vi "PID Veering.vi"(6 "Deviation":dbl, 7 "Current Distance":dbl=15.0 format="%#_13g", 8 "error in (no error)":errorcluster, 11 "Refnum's":T1={"Gyro"="Gyro", "Mtr 1"="LeftMtr", "Mtr 2"="RightMtr"}) -> (0 "error out":errorcluster)   [LabVIEW 2017]
uses:
  <vilib>/addons/control/pid/pid.llb/PID (DBL).vi
  <vilib>/addons/control/pid/NI_PID_pid.lvlib
panel:
  out "Right":dbl
  out "Left":dbl
  in  "V-D":dbl format="%#_13g"
  in  "V-I":dbl format="%#_13g"
  in  "V-P":dbl=0.01 format="%#_13g"
  in  "D-D":dbl format="%#_13g"
  in  "D-I":dbl format="%#_13g"
  in  "D-P":dbl=0.02 format="%#_13g"
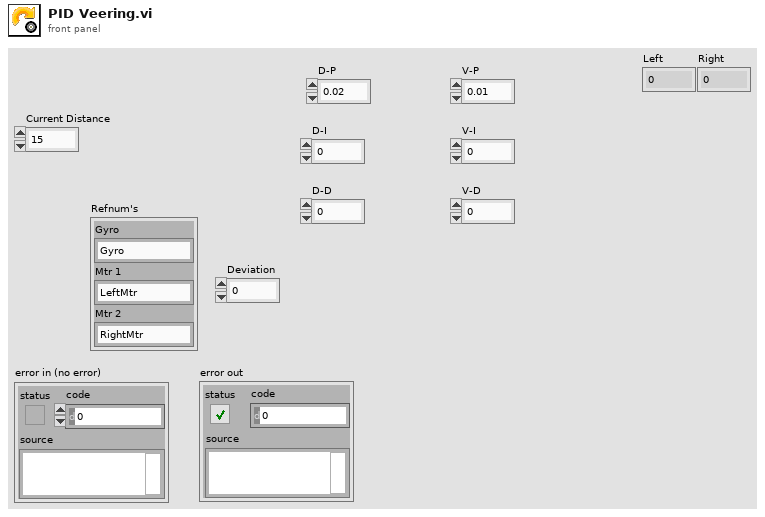
[diagram p1: front panel]
types:
  T1 = cluster{"Gyro":string, "Mtr 1":string, "Mtr 2":string}
  T2 = typedef "WPI_MotorControlDeviceRef.ctl" = cluster{"DeviceStatus":errorcluster, "Type":T3, "PWM":cluster{"PWM Channel":T4, "DeadBand":T5}, "CAN":cluster{"Device Number":u8, "SetOutput VI Ref":variant, "GetOutput VI Ref":variant, "Enable VI Ref":variant, "Disable VI Ref":variant, "Data":variant}, "Invert":bool, "DIO PWM":cluster{"PWM \"Enable\" Channel":T4, "DIOChannel":T6, "PWM Rate":dbl}}
  T3 = typedef "WPI_MotorControlType.ctl" = enum16{"PWM", "CAN", "DIO PWM"}
  T4 = typedef "FPGA_DIOPWMChannel.ctl" = enum8{"PWM 0", "PWM 1", "PWM 2", "PWM 3", "PWM 4", "PWM 5", "PWM 6", "PWM 7", "PWM 8", "PWM 9", "PWM MXP 0", "PWM MXP 1", "PWM MXP 2", "PWM MXP 3", "PWM MXP 4", "PWM MXP 5", "PWM MXP 6", "PWM MXP 7", "PWM MXP 8", "PWM MXP 9", "Invalid"}
  T5 = typedef "WPI_PWMDeadband.ctl" = cluster{"Name":string, "maxPositivePwm":i32, "minPositivePwm":i32, "centerPwm":i32, "maxNegativePwm":i32, "minNegativePwm":i32, "angularRange":u16}
  T6 = typedef "FPGA_DIOChannel.ctl" = enum8{"DIO 0", "DIO 1", "DIO 2", "DIO 3", "DIO 4", "DIO 5", "DIO 6", "DIO 7", "DIO 8", "DIO 9", "DIO MXP 0", "DIO MXP 1", "DIO MXP 2", "DIO MXP 3", "DIO MXP 4", "DIO MXP 5", "DIO MXP 6", "DIO MXP 7", "DIO MXP 8", "DIO MXP 9", "DIO MXP 10", "DIO MXP 11", "DIO MXP 12", "DIO MXP 13", "DIO MXP 14", "DIO MXP 15", "SPI Port CS1", "SPI Port CS2", "SPI Port CS3", "SPI Port MISO", "SPI Port MOSI", "Invalid"}
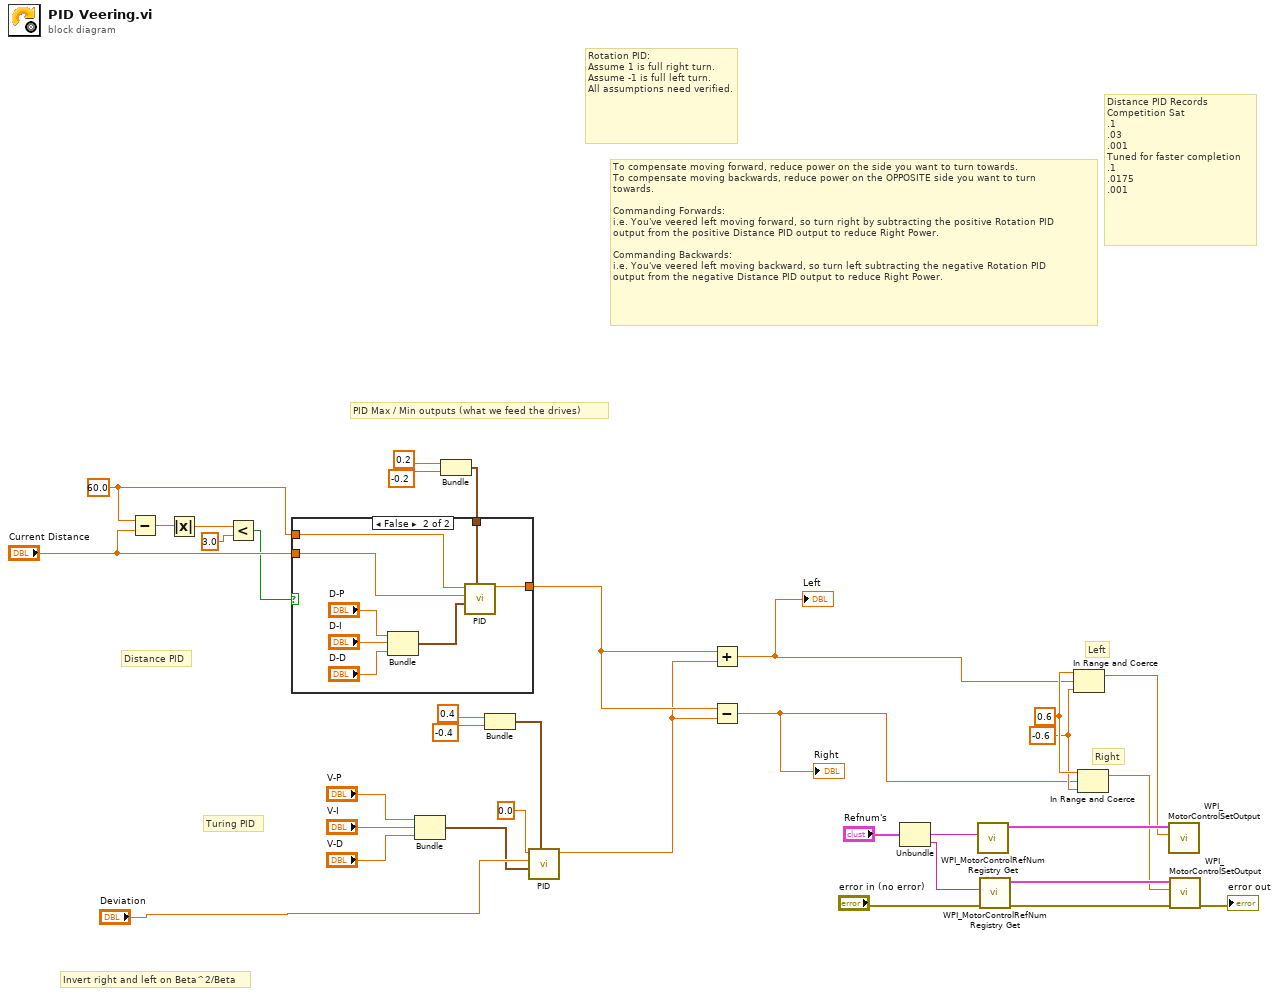
[diagram p0: block diagram]
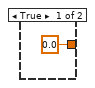
[diagram p2: hidden frame]
diagram:
  w13 = 60.0 ("setpoint")
  w28 = -0.6
  w29 = 0.6
  # "Right"
  # "Left"
  # "Turing PID"
  # "Distance PID"
  # "Distance PID Records\nCompetition Sat\n.1\n.03\n.001\nTuned for faster completion\n.1\n.0175\n.001"
  # "Invert right and left on Beta^2/Beta"
  # "To compensate moving forward, reduce power on the side you want to turn towards.\nTo compensate moving backwards, reduce power on the OPPOSITE side you want to turn\ntowards.\n\nCommanding Forwards:\ni.e. You've veered left moving forward, so turn right by subtracting the positive Rotation PID\noutput from the positive Distance PID output to reduce Right Power.\n\nCommanding Backwards:\ni.e. You've veered left moving backward, so turn left subtracting the negative Rotation PID \noutput from the negative Distance PID output to reduce Right Power."
  # "PID Max / Min outputs (what we feed the drives)"
  # "Rotation PID:\nAssume 1 is full right turn.\nAssume -1 is full left turn.\nAll assumptions need verified."
  n1 = Subtract(x=w13, y="Current Distance") -> (x-y=w11:dbl)
  n2 = Absolute Value(x=w11) -> (abs(x)=w14:dbl)
  n3 = Less?(x=w14, y=3.0) -> (x < y?=w10:bool)
  n4 = Bundle("V-P"="V-P", "V-I"="V-I", "V-D"="V-D") -> (w2:cluster{"V-P":dbl, "V-I":dbl, "V-D":dbl})  [unwired: 1 in]
  n5 = Bundle(0.2, -0.2) -> (w30:cluster{dbl, dbl})  [unwired: 1 in]
  n6 = case shown="False" w10 {
    tunnel: w30 -> [_ w39]
    tunnel: "Current Distance" -> [_ w38]
    tunnel: [0.0 ("output") w37] -> w9
    tunnel: w13 -> [_ w36]
    frame True {
    }
    frame False {
      n7 = Bundle("D-P"="D-P", "D-I"="D-I", "D-D"="D-D") -> (w40:cluster{"D-P":dbl, "D-I":dbl, "D-D":dbl})  [unwired: 1 in]
      n8 = call-poly <vilib>:"PID.vi"("output range"=w39, "PID gains"=w40, "process variable"=w38, "setpoint"=w36) -> ("output"=w37:dbl)  [unwired: 6 in, 1 out]
    }
  }
  n9 = Bundle(0.4, -0.4) -> (w16:cluster{dbl, dbl})  [unwired: 1 in]
  n10 = call-poly <vilib>:"PID.vi"("output range"=w16, "PID gains"=w2, "process variable"="Deviation", "setpoint"=0.0) -> ("output"=w8:dbl)  [unwired: 6 in, 1 out]
  n11 = Add(x=w9, y=w8) -> (x+y=w6:dbl)
  "Left" <- w6
  n12 = Subtract(x=w9, y=w8) -> (x-y=w7:dbl)
  "Right" <- w7
  n13 = Unbundle("Refnum's") -> ("Mtr 1"=w34:string, "Mtr 2"=w33:string)  [unwired: 1 out]
  n14 = call <vilib>:"WPI_MotorControlRefNum Registry Get.vi"("refnum name"=w34) -> ("MotorControlDevRef"=w25:T2)  [unwired: 9 in, 1 out]
  n15 = call <vilib>:"WPI_MotorControlRefNum Registry Get.vi"("error in (no error)"="error in (no error)", "refnum name"=w33) -> ("error out"=w20:errorcluster, "MotorControlDevRef"=w26:T2)  [unwired: 8 in]
  n16 = In Range and Coerce(upper limit=w29, x=w6, lower limit=w28) -> (coerced(x)=w24:dbl)  [unwired: 1 out]
  n17 = In Range and Coerce(upper limit=w29, x=w7, lower limit=w28) -> (coerced(x)=w23:dbl)  [unwired: 1 out]
  n18 = call <vilib>:"WPI_MotorControlSetOutput.vi"("Output"=w24, "MotorControlDevRef"=w25) -> ()  [unwired: 7 in, 3 out]
  n19 = call <vilib>:"WPI_MotorControlSetOutput.vi"("error in (no error)"=w20, "Output"=w23, "MotorControlDevRef"=w26) -> ("error out"=→"error out":errorcluster)  [unwired: 6 in, 2 out]
